vi "LogONSD.vi"(3 "error in (no error)":errorcluster, 4 "Real delay time, ps":dbl, 5 "Experiment in":refnum<class "Experiment.lvclass">) -> (0 "error out":errorcluster, 1 "String":string, 2 "Path":path)   [LabVIEW 2015]
uses:
  Classes/Experiment.lvclass
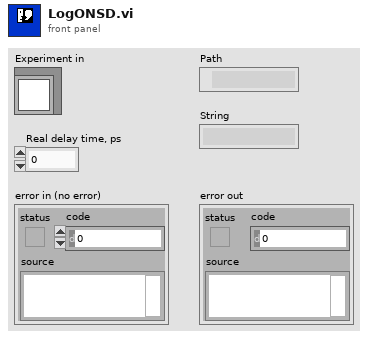
[diagram p1: front panel]
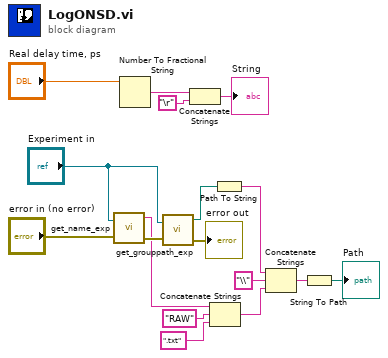
[diagram p0: block diagram]
diagram:
  n1 = call-dynamic "get_name_exp.vi"("Experiment.lvclass in"="Experiment in", "error in (no error)"="error in (no error)") -> ("Exp name"=w9:string, "error out"=w16:errorcluster)  [unwired: 1 out]
  n2 = Number To Fractional String(number="Real delay time, ps") -> (F-format string=w3:string)  [unwired: 3 in]
  n3 = call-dynamic "get_grouppath_exp.vi"("Experiment.lvclass in"="Experiment in", "error in (no error)"=w16) -> ("GroupPath"=w14:path, "error out"=→"error out":errorcluster)  [unwired: 1 out]
  n4 = Concatenate Strings(w3, "\r") -> (→"String":string)
  n5 = Concatenate Strings(w9, "RAW" ("string"), ".txt" ("string")) -> (w7:string)
  n6 = Path To String(path=w14) -> (string=w6:string)
  n7 = Concatenate Strings(w6, "\\" ("string"), w7) -> (w12:string)
  n8 = String To Path(string=w12) -> (path=→"Path":path)
